vi "KalmanFilter_SetXHat_Single.vi"(9 "xHat":dbl, 10 "Row":i32, 11 "in KalmanFilter":T1) -> (0 "Error":bool, 3 "out KalmanFilter":T1)   [LabVIEW 2019, in "Trajectory_Library.lvlib"]
doc: "Creates a new LINEAR SYSTEM data cluster with the specified values. \n\n\nInputs: \n - XXX -- XXX.\n\nOutputs:\n - XXX -- XXX."
uses:
  Trajectory_Library.lvlib
  KALMAN_FILTER.ctl
  <vilib>/Analysis/Matrix/Datatypes/RealMatrix.ctl
  LINEAR_SYSTEM.ctl
  <vilib>/Analysis/Matrix/NI_Matrix.lvlib
panel:
  # "Steady State Gain  \n<States,Outputs>"
  # "State Estimate <Statess,1>"
  # "<States,States>"
  # "<States,Inputs>"
  # "<Outputs,States>"
  # "<Outputs,Inputs>"
  # "Steady State Gain  \n<States,Outputs>"
  # "State Estimate <Statess,1>"
  # "<States,States>"
  # "<States,Inputs>"
  # "<Outputs,States>"
  # "<Outputs,Inputs>"
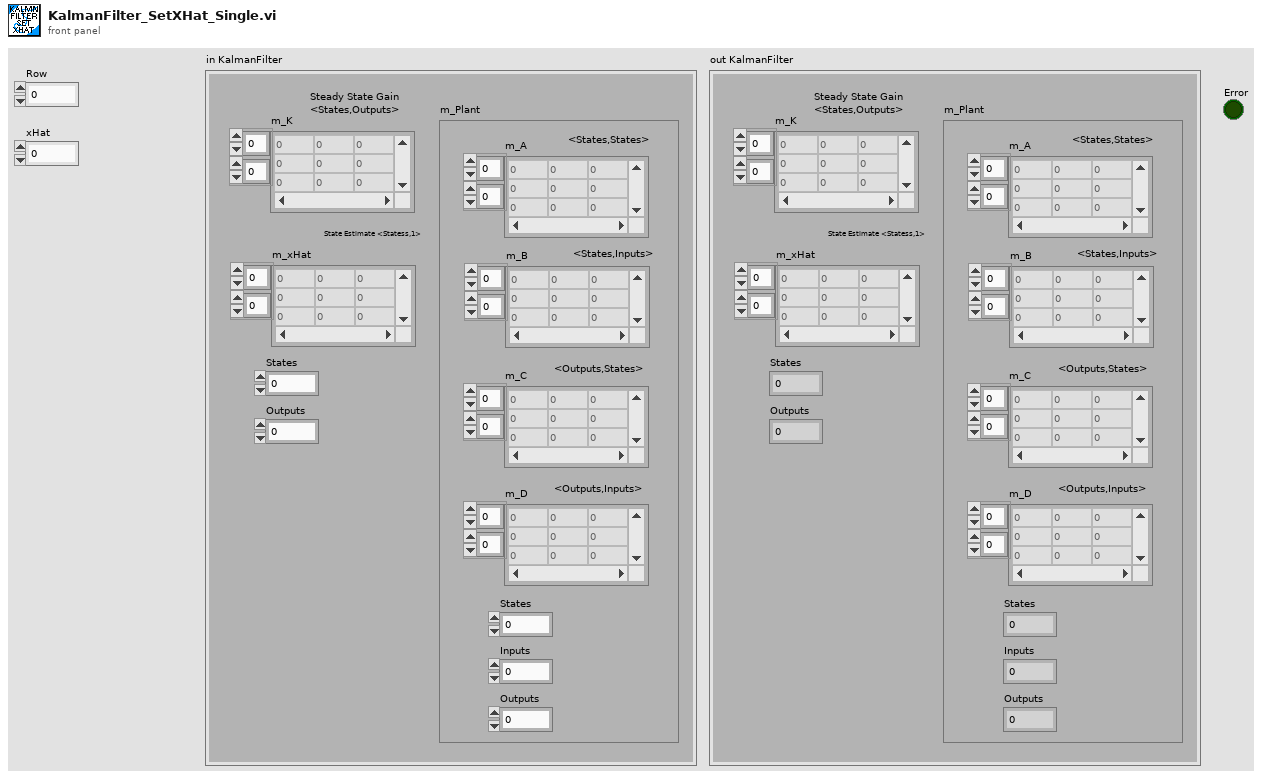
[diagram p1: front panel]
types:
  T1 = typedef "Trajectory_Library.lvlib/KALMAN_FILTER.ctl" = cluster{"m_K":T2, "m_xHat":T2, "States":i32, "Outputs":i32, "m_Plant":T3}
  T2 = typedef "NI_Matrix.lvlib/RealMatrix.ctl" = dbl[][]
  T3 = typedef "Trajectory_Library.lvlib/LINEAR_SYSTEM.ctl" = cluster{"m_A":T2, "m_B":T2, "m_C":T2, "m_D":T2, "States":i32, "Inputs":i32, "Outputs":i32}
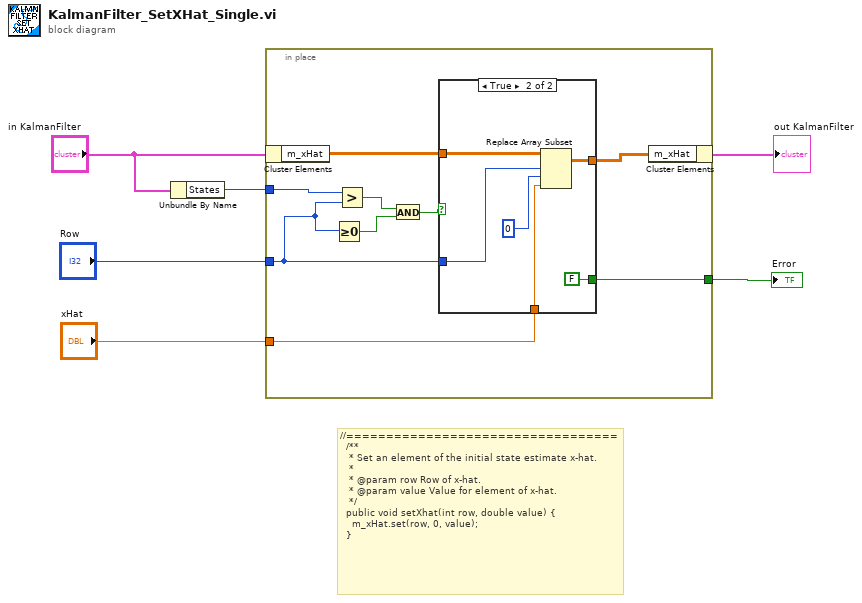
[diagram p0: block diagram]
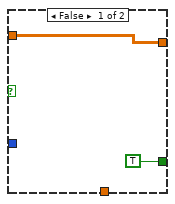
[diagram p2: hidden frame]
diagram:
  # "//==================================\n  /**\n   * Set an element of the initial state estimate x-hat.\n   *\n   * @param row Row of x-hat.\n   * @param value Value for element of x-hat.\n   */\n  public void setXhat(int row, double value) {\n    m_xHat.set(row, 0, value);\n  }"
  n1 = Unbundle By Name("in KalmanFilter") -> ("States"=w6:i32)
  n2 = in-place {
    in-place-border: "Row" -> [w9]
    in-place-border: "xHat" -> [w13]
    in-place-border: w6 -> [w10]
    in-place-border: [w7] -> w1
    n3 = in-place-cluster #1("in KalmanFilter") -> ("m_xHat"=w15:T2)
    n4 = Greater Or Equal To 0?(x=w9) -> (x >= 0?=w11:bool)
    n5 = Greater?(x=w10, y=w9) -> (0:w12:bool)
    n6 = And(x=w12, y=w11) -> (x .and. y?=w8:bool)
    n7 = case shown="True" w8 {
      tunnel: w15 -> [w17 w23]
      tunnel: [w17 w22] -> w14
      tunnel: w13 -> [_ w20]
      tunnel: w9 -> [_ w19]
      tunnel: [TRUE FALSE] -> w7
      frame False {
      }
      frame True {
        n8 = Replace Array Subset(array=w23, new element=w20, index (row)=w19, index (col)=0) -> (w22:T2)
      }
    }
    n9 = in-place-cluster #1("m_xHat"=w14) -> (→"out KalmanFilter":T1)
  }
  "Error" <- w1
